vi "Scale Start-End Distance.vi"(7 "Distance Format":u8, 10 "End Distance":dbl, 11 "Start Distance":dbl) -> (3 "Start-End Scaled":dbl[](array[numeric]))   [LabVIEW 2024]
uses:
  Modules/POSCONV/POSCONV.lvlib
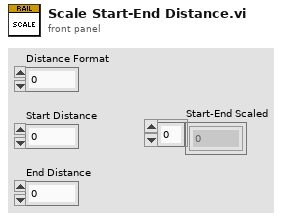
[diagram p1: front panel]
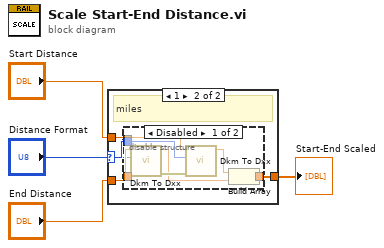
[diagram p0: block diagram]
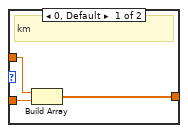
[diagram p2: hidden frame]
diagram:
  n1 = case shown="1" "Distance Format" {
    selector: "Distance Format" -> [_ w8]
    tunnel: "End Distance" -> [w7 w10]
    tunnel: "Start Distance" -> [w6 w9]
    tunnel: [w5 w11] -> w3
    frame 0, Default {
      # "km"
      n2 = Build Array(w6, w7) -> (w5:dbl[])
    }
    frame 1 {
      # "miles"
      n3 = disable-structure shown="Disabled" {
        disable-tunnel: [w18 _] -> w11
        disable-tunnel: w10 -> [w16 _]
        disable-tunnel: w9 -> [w15 _]
        disable-tunnel: w8 -> [w12 _]
        frame Disabled {
          n4 = call "Dkm To Dxx.vi"("units"=w12, "dKilo"=w16) -> ("error out"=w17:errorcluster, "dXX_Converted"=w14:dbl)  [unwired: 8 in]
          n5 = call "Dkm To Dxx.vi"("error in (no error)"=w17, "units"=w12, "dKilo"=w15) -> ("dXX_Converted"=w13:dbl)  [unwired: 7 in, 1 out]
          n6 = Build Array(w13, w14) -> (w18:dbl[])
        }
        frame Enabled {
        }
      }
    }
  }
  "Start-End Scaled" <- w3
